vi "Get Parameter Value - String.vi"(7 "Default value":string, 8 "error in (no error)":errorcluster, 9 "Parameter name":string, 10 "Config name":string, 11 "Config in":refnum<class "Config.lvclass">) -> (0 "error out":errorcluster, 2 "Value":string, 3 "Config out":refnum<class "Config.lvclass">)   [LabVIEW 2026, in "TALOS.lvlib" / "Classes.lvlib" / "Config.lvclass"]
doc: "Get the parameter's value (string) from the specified configuration. Use the data type terminal to specify the output type."
uses:
  Config.lvclass
  Config.lvclass/Config.ctl
  Ancestor/Ancestor/Ancestor.lvclass/Ancestor.ctl
  FGV/Error Memory/Get Error Description.vi
  Support VIs/Get PC name.vi
  Ancestor/Ancestor/Read ID.vi
  Support VIs/Get Class Name.vi
  <vilib>/Utility/error.llb/Clear Errors.vi
  FGV/Error Memory/Error Memory Core.vi
  <vilib>/AdvancedString/Delimited String to 1D String Array.vi
  <vilib>/AdvancedString/Delimited String to 1D String Array (string).vi
  Support VIs/Circus Root Path.vi
  FGV/Error Memory/Error Crt Lvl checker.vi
  FGV/Error Memory/Error Memory Core.vi/40c8088d-b597-4017-91af-faa98e00292e.vi
  FGV/Error Memory/Error Memory Core.vi/d4a3ab98-063c-4e44-b43d-fbdcfe6c2be2.vi
  Support VIs/Global Memory.vi
  <vilib>/Utility/LVClass/Get LV Class Name.vi
  Support VIs/Is in Packed Library.vi
  Support VIs/TALOS Root path.vi
  Support VIs/Read CSV worksheet.vi
  Support VIs/Global Constants.vi
  <vilib>/Utility/error.llb/General Error Handler.vi
  Ancestor/Ancestor/Ancestor.lvclass
  <vilib>/Comparison/Equal/Equal Functor/Equal Functor.lvclass
  TALOS.lvlib
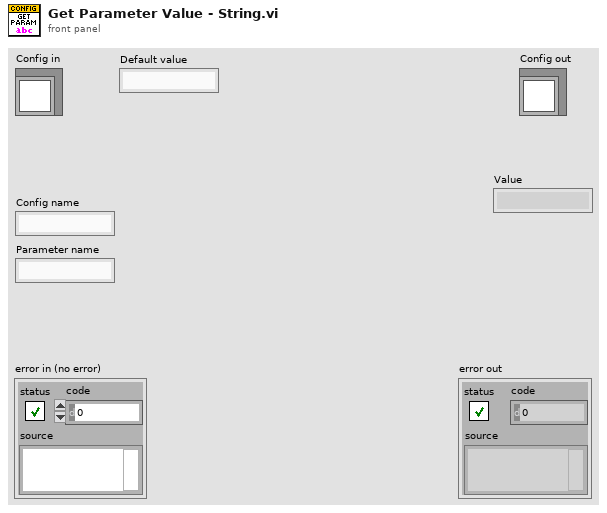
[diagram p1: front panel]
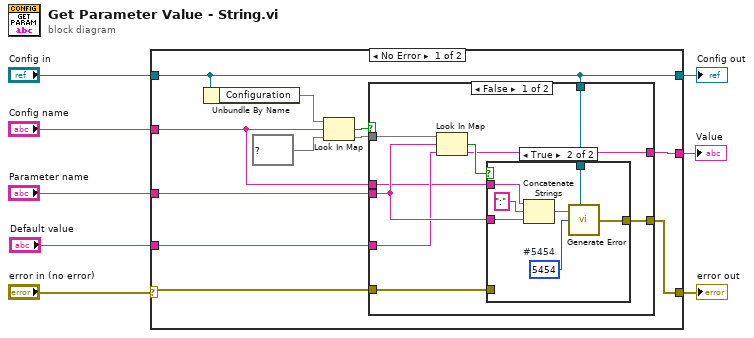
[diagram p0: block diagram]
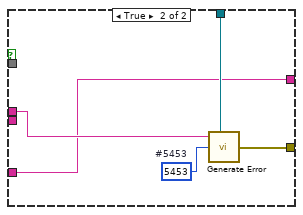
[diagram p3: hidden frame]
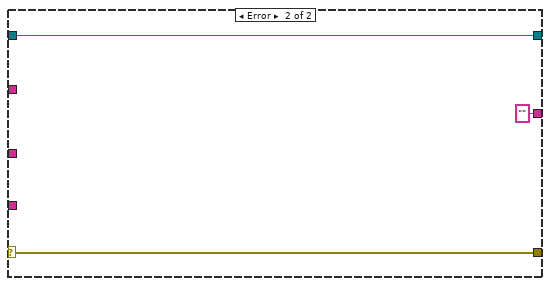
[diagram p4: hidden frame]
diagram:
  n1 = case shown="No Error" "error in (no error)" {
    selector: "error in (no error)" -> [w9 w44]
    tunnel: [w16 w44] -> w2
    tunnel: [w13 w43] -> w4
    tunnel: "Config in" -> [w13 w43]
    tunnel: "Parameter name" -> [w17 _]
    tunnel: [w14 "" ("Value")] -> w3
    tunnel: "Config name" -> [w12 _]
    tunnel: "Default value" -> [w10 _]
    frame No Error {
      n2 = Unbundle By Name(w13) -> ("Configuration"=w19:map{string, map{string, string}})
      n3 = Look In Map(map=w19, key=w12, default value=map{string, string} {}) -> (key not found?=w15:bool, value=w18:map{string, string})
      n4 = case shown="False" w15 {
        tunnel: w12 -> [w20 w39]
        tunnel: w18 -> [w26 _]
        tunnel: w17 -> [w25 _]
        tunnel: [w27 w40] -> w16
        tunnel: [w21 w37] -> w14
        tunnel: w13 -> [w28 w38]
        tunnel: w10 -> [w22 w37]
        tunnel: w9 -> [w23 _]
        frame False {
          n5 = Look In Map(map=w26, key=w25, default value=w22) -> (key not found?=w24:bool, value=w21:string)
          n6 = case shown="True" w24 {
            tunnel: w28 -> [_ w35]
            tunnel: [w29 w36] -> w27
            tunnel: w25 -> [_ w32]
            tunnel: w23 -> [w29 _]
            tunnel: w20 -> [_ w33]
            frame False {
            }
            frame True {
              w34 = 5454  # #5454
              n7 = Concatenate Strings(w33, ":" ("string"), w32) -> (w30:string)
              n8 = call "Generate Error.vi"("Optional String"=w30, "Class"=w35, "Error Code"=w34) -> ("error out"=w36:errorcluster)  [unwired: 4 in]
            }
          }
        }
        frame True {
          w41 = 5453  # #5453
          n9 = call "Generate Error.vi"("Optional String"=w39, "Class"=w38, "Error Code"=w41) -> ("error out"=w40:errorcluster)  [unwired: 4 in]
        }
      }
    }
    frame Error {
    }
  }
  "error out" <- w2
  "Config out" <- w4
  "Value" <- w3
